vi "init.vi"(8 "error in (no error)":errorcluster {"code" format="%x"}, 9 "com_port":string, 10 "type":u16(ring)=65535 items=["XC_120PC"=0, "XC_exacte"=1, "XC_120LED"=2, "XC_110LED"=3, "XC_mini"=4, "XC_XYLIS"=5, "XC_XR210"=6, "XC_LED1"=7, "XC_XT600"=8, "XC_XT900"=9, "Any"=65535], 11 "Xcite in":refnum<class "Xcite.lvclass">) -> (0 "error out":errorcluster, 3 "Xcite out":refnum<class "Xcite.lvclass">)   [LabVIEW 2019, in "Xcite.lvclass"]
doc: "Searches for XCite devices on the system comm ports. Device type and comm port to search can be specified. If not specified, all devices and comm ports are searched."
uses:
  Xcite.lvclass
  Xcite.lvclass/Xcite.ctl
  etc.xcite/XCite.lvlib
panel:
  out "found_type":u16
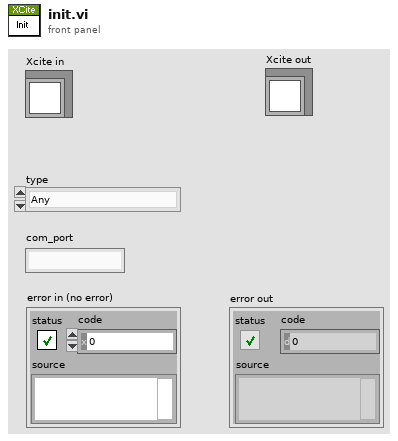
[diagram p1: front panel]
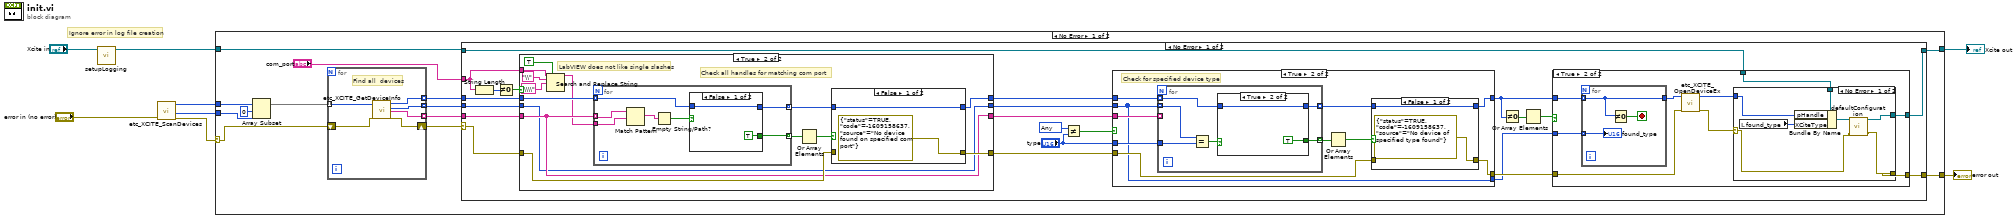
[diagram p0: block diagram]
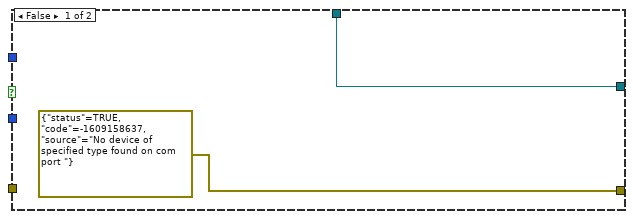
[diagram p2: hidden frame]
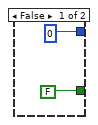
[diagram p6: hidden frame]
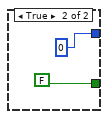
[diagram p9: hidden frame]
diagram:
  # "Ignore error in log file creation"
  n1 = call "setupLogging.vi"("Xcite in"="Xcite in") -> ("Xcite out"=w1:refnum<class "Xcite.lvclass">)  [unwired: 9 in, 1 out]
  n2 = call "etc_XCITE_ScanDevices.vi"("error in (no error)"="error in (no error)") -> ("error out"=w6:errorcluster, "buf_len_out"=w3:u32, "ph out"=w7:u64[])  [unwired: 7 in, 1 out]
  n3 = case shown="No Error" w6 {
    selector: w6 -> [w18 w136]
    tunnel: w7 -> [w21 _]
    tunnel: w3 -> [w20 _]
    tunnel: [w11 w136] -> w5
    tunnel: w1 -> [w10 w135]
    tunnel: [w9 w135] -> w4
    frame No Error {
      n4 = Array Subset(array=w21, index=0, length=w20) -> (w17:u64[])
      n5 = for {
        tunnel: w17 -> [w133] mode=indexing
        tunnel: [w132] -> w13 mode=indexing
        tunnel: [w129] -> w14 mode=indexing
        tunnel: [w131] -> w15 mode=indexing
        shift-right: [w130] -> w16
        shift-left: w18 -> [w134]
        # "Find all  devices"
        n6 = call "etc_XCITE_GetDeviceInfo.vi"("h"=w133, "error in (no error)"=w134) -> ("h out"=w132:u64, "type"=w129:i32, "port"=w131:string, "error out"=w130:errorcluster)  [unwired: 12 in, 2 out]
      }
      n7 = case shown="No Error" w16 {
        selector: w16 -> [w37 w128]
        tunnel: "com_port" -> [w41 _]
        tunnel: w15 -> [w40 _]
        tunnel: w14 -> [w39 _]
        tunnel: w13 -> [w38 _]
        tunnel: [w25 w128] -> w11
        tunnel: w10 -> [w24 w127]
        tunnel: [w23 w127] -> w9
        frame No Error {
          w36 = u16 65535 items=["XC_120PC"=0, "XC_exacte"=1, "XC_120LED"=2, "XC_110LED"=3, "XC_mini"=4, "XC_XYLIS"=5, "XC_XR210"=6, "XC_LED1"=7, "XC_XT600"=8, "XC_XT900"=9, "Any"=65535] ("XCiteType")
          n8 = String Length(string=w41) -> (length=w43:i32)
          n9 = Not Equal To 0?(x=w43) -> (x != 0?=w42:bool)
          n10 = case shown="True" w42 {
            tunnel: w41 -> [_ w101]
            tunnel: w40 -> [w96 w106]
            tunnel: w39 -> [w95 w103]
            tunnel: w38 -> [w94 w105]
            tunnel: w37 -> [w97 w108]
            tunnel: [w97 w107] -> w30
            tunnel: [w96 w106] -> w32
            tunnel: [w95 w103] -> w33
            tunnel: [w94 w104] -> w34
            frame False {
              # "Com port not specified."
            }
            frame True {
              # "LabVIEW does not like single slashes"
              # "Check all handles for matching com port"
              n11 = Search and Replace String(replace all?=TRUE ("replace all? (F)"), input string=w101, search string="\\", replace string="\\\\" ("replace string (\"\")")) -> (result string=w102:string)  [unwired: 4 in, 3 out]
              n12 = for {
                tunnel: w105 -> [w118] mode=indexing
                tunnel: w106 -> [w122] mode=indexing
                tunnel: w102 -> [w121]
                tunnel: [w117] -> w109 mode=indexing
                tunnel: [w116] -> w111 mode=indexing
                n13 = Match Pattern(string=w122, regular expression=w121) -> (match substring=w120:string)  [unwired: 1 in, 3 out]
                n14 = Empty String/Path?(string/path=w120) -> (empty?=w119:bool)
                n15 = case shown="False" w119 {
                  tunnel: [w124 u64 0] -> w117
                  tunnel: w118 -> [w124 _]
                  tunnel: [TRUE FALSE] -> w116
                  frame False {
                  }
                  frame True {
                  }
                }
              }
              n16 = Or Array Elements(Boolean array=w111) -> (logical OR=w110:bool)
              n17 = case shown="False" w110 {
                tunnel: w109 -> [w113 w115]
                tunnel: [w113 w115] -> w104
                tunnel: w108 -> [_ w114]
                tunnel: [errorcluster {"status"=TRUE, "code"=-1609158637, "source"="No device found on specified com port"} ("error IO") w114] -> w107
                frame False {
                }
                frame True {
                }
              }
            }
          }
          n18 = Not Equal?(x=w36, y="type") -> (x != y?=w35:bool)
          n19 = case shown="True" w35 {
            tunnel: w34 -> [w68 w79]
            tunnel: w33 -> [w67 w70]
            tunnel: w32 -> [_ w78]
            tunnel: "type" -> [_ w77]
            tunnel: w30 -> [w69 w73]
            tunnel: [w69 w72] -> w26
            tunnel: [w68 w71] -> w27
            tunnel: [w67 w70] -> w22
            frame False {
            }
            frame True {
              # "Check for specified device type"
              n20 = for {
                tunnel: w79 -> [w86] mode=indexing
                tunnel: w70 -> [w88] mode=indexing
                tunnel: w78 -> [_] mode=indexing
                tunnel: w77 -> [w89]
                tunnel: [w85] -> w74 mode=indexing
                tunnel: [w84] -> w76 mode=indexing
                n21 = Equal?(x=w88, y=w89) -> (x = y?=w87:bool)
                n22 = case shown="True" w87 {
                  tunnel: w86 -> [_ w93]
                  tunnel: [u64 0 w93] -> w85
                  tunnel: [FALSE TRUE] -> w84
                  frame False {
                  }
                  frame True {
                  }
                }
              }
              n23 = Or Array Elements(Boolean array=w76) -> (logical OR=w75:bool)
              n24 = case shown="False" w75 {
                tunnel: w74 -> [w80 w82]
                tunnel: w73 -> [_ w83]
                tunnel: [errorcluster {"status"=TRUE, "code"=-1609158637, "source"="No device of specified type found"} ("error IO") w83] -> w72
                tunnel: [w80 w82] -> w71
                frame False {
                }
                frame True {
                }
              }
            }
          }
          n25 = Not Equal To 0?(x=w27) -> (x != 0?=w29:bool[])
          n26 = Or Array Elements(Boolean array=w29) -> (logical OR=w28:bool)
          n27 = case shown="True" w28 {
            tunnel: w27 -> [_ w54]
            tunnel: w26 -> [_ w52]
            tunnel: [errorcluster {"status"=TRUE, "code"=-1609158637, "source"="No device of specified type found on com port "} ("error IO") w50] -> w25
            tunnel: w24 -> [w44 w49]
            tunnel: [w44 w47] -> w23
            tunnel: w22 -> [_ w46]
            frame False {
            }
            frame True {
              n28 = for {
                tunnel: w54 -> [w66] mode=indexing
                tunnel: [w66] -> w53
                tunnel: w46 -> [w64] mode=indexing
                stop <- w65 stop-if-true
                n29 = Not Equal To 0?(x=w66) -> (x != 0?=w65:bool)
                "found_type" <- w64
              }
              n30 = call "etc_XCITE_OpenDeviceEx.vi"("error in (no error)"=w52, "h"=w53) -> ("error out"=w51:errorcluster, "h out"=w48:u64)  [unwired: 7 in, 1 out]
              n31 = case shown="No Error" w51 {
                selector: w51 -> [w57 w63]
                tunnel: [w56 w63] -> w50
                tunnel: w49 -> [w61 w62]
                tunnel: w48 -> [w60 _]
                tunnel: [w55 w62] -> w47
                frame No Error {
                  n32 = local read "found_type"() -> (w59:u16)
                  n33 = Bundle By Name(cluster=w61, "pHandle"=w60, "XCiteType"=w59) -> (w58:refnum<class "Xcite.lvclass">)
                  n34 = call "defaultConfiguration.vi"("error in (no error)"=w57, "Xcite in"=w58) -> ("error out"=w56:errorcluster, "Xcite out"=w55:refnum<class "Xcite.lvclass">)  [unwired: 8 in]
                }
                frame Error {
                }
              }
            }
          }
        }
        frame Error {
        }
      }
    }
    frame Error {
    }
  }
  "Xcite out" <- w4
  "error out" <- w5
